vi "Initialization VI Name.vi"(11 "CD Template in":refnum<class "NIVS_CD Template.lvclass">) -> (2 "Initialization VI Name":string)   [LabVIEW 2017, in "NIVS_CD Template.lvclass"]
uses:
  NIVS_CD Template.lvclass
  NIVS_Consolidated_CDW_MetaDataObj/CD System Explorer lvlib.ctl
  NIVS_Consolidated_CDW_MetaDataObj/CD System Explorer lvlib.vi
  NIVS_Consolidated_CDW_MetaDataObj/NIVS_Consolidated_CDW_MetaDataObj.lvclass
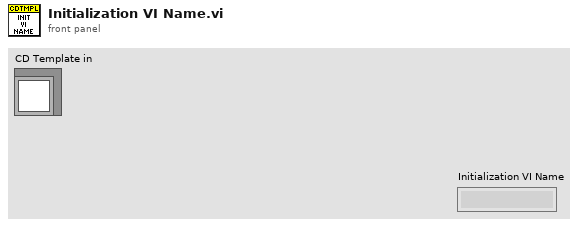
[diagram p1: front panel]
types:
  T1 = typedef "NIVS_Consolidated_CDW_MetaDataObj.lvclass/CD System Explorer lvlib.ctl" = enum16{"LibraryFileName", "LibraryFolderName", "System Explorer.FolderName", "System Explorer.Dynamically Called.FolderName", "System Explorer.Dynamically Called.Extra Pages.FolderName", "System Explorer.Dynamically Called.Extra Pages.TemplatePathAndName", "System Explorer.Dynamically Called.Main Page.VIName", "System Explorer.Dynamically Called.Main Page.TemplatePathAndName", "System Explorer.Dynamically Called.Initialization VI.VIName", "System Explorer.Dynamically Called.Initialization VI.TemplatePathAndName", "System Explorer.SubVI.FolderName", "System Explorer.Types.FolderName", "System Explorer.ActionVIOnCompile.VIName", "System Explorer.ExportConfigRTM.VIName", "System Explorer.LoadHelpFile.VIName"}
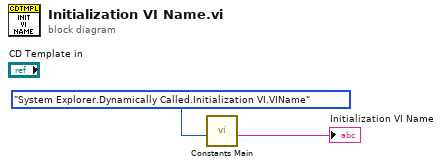
[diagram p0: block diagram]
diagram:
  n1 = call-poly "Constants Main.vi"("Action"=CD_System_Explorer_lvlib."System Explorer.Dynamically Called.Initialization VI.VIName") -> ("Output"=→"Initialization VI Name":string)  [unwired: 10 in]
